vi "WriteData.vi"(8 "error in":errorcluster, 11 "refnum in":refnum<file>) -> (0 "error out":errorcluster, 3 "refnum out":refnum<file>)   [LabVIEW 2017]
doc: "Logs data to csv file on roborio"
uses:
  <vilib>/Rock Robotics/Network Tables/NT Read Number.vi
  <vilib>/Rock Robotics/Network Tables/NT Read Boolean.vi
  <vilib>/Rock Robotics/Network Tables/NT Read String.vi
  Robot Global Data.vi
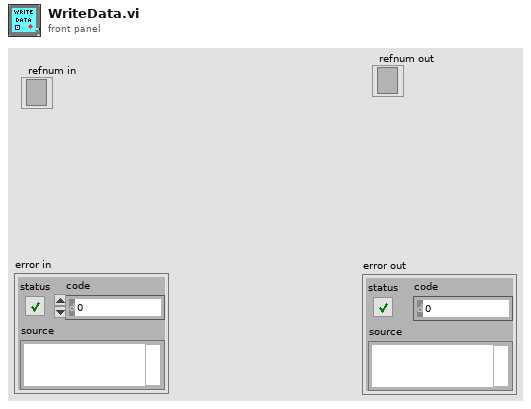
[diagram p1: front panel]
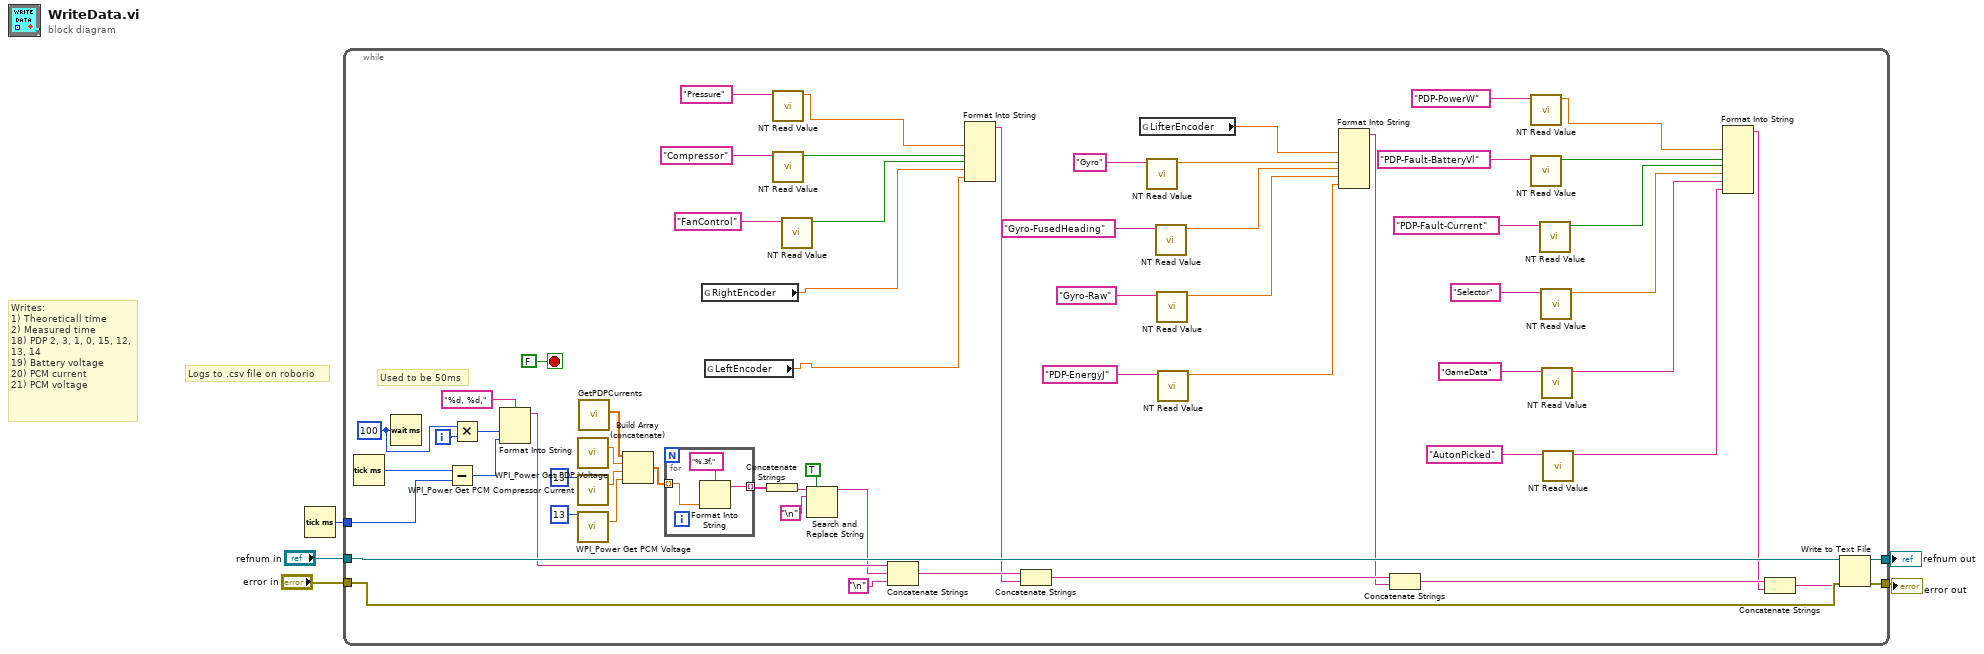
[diagram p0: block diagram]
diagram:
  # "Logs to .csv file on roborio"
  # "Writes:\n1) Theoreticall time\n2) Measured time\n18) PDP 2, 3, 1, 0, 15, 12,\n13, 14\n19) Battery voltage\n20) PCM current\n21) PCM voltage"
  n1 = Tick Count (ms)() -> (millisecond timer value=w1:u32)
  n2 = while {
    tunnel: "error in" -> [w65]
    tunnel: "refnum in" -> [w64]
    tunnel: [w62] -> w3
    tunnel: [w63] -> w2
    tunnel: w1 -> [w61]
    i -> [w66]
    stop <- FALSE stop-if-true
    w60 = u32 100 ("milliseconds to wait")
    # "Used to be 50ms"
    n3 = Tick Count (ms)() -> (millisecond timer value=w48:u32)
    n4 = Wait (ms)(milliseconds to wait=w60) -> ()  [unwired: 1 out]
    n5 = Subtract(x=w48, y=w61) -> (x-y=w47:u32)
    n6 = Multiply(x=w60, y=w66) -> (x*y=w59:u32)
    n7 = Format Into String(format string="%d, %d,", w59, w47) -> (resulting string=w44:string)  [unwired: 2 in, 1 out]
    n8 = call <vilib>:"WPI_Power Get PDP Voltage.vi"() -> ("voltage (V)"=w55:dbl)  [unwired: 14 in, 1 out]
    n9 = call <vilib>:"WPI_Power Get PCM Compressor Current.vi"("Pneumatics Control Module (0)"=u8 13) -> ("current (A)"=w51:dbl)  [unwired: 13 in, 1 out]
    n10 = call <vilib>:"WPI_Power Get PCM Voltage.vi"("Pneumatics Control Module (0)"=u8 13) -> ("Input Voltage"=w50:dbl)  [unwired: 12 in, 2 out]
    n11 = call "GetPDPCurrents.vi"() -> ("PDP Currents"=w49:dbl[])  [unwired: 11 in]
    n12 = Build Array (concatenate)(w49, w55, w51, w50) -> (w54:dbl[])
    n13 = for {
      tunnel: w54 -> [w70] mode=indexing
      tunnel: [w68] -> w53 mode=indexing
      n14 = Format Into String(format string="%.3f,", w70) -> (resulting string=w68:string)  [unwired: 2 in, 1 out]
    }
    n15 = global read "Robot Global Data.vi" "RightEncoder"() -> (w6:dbl)
    n16 = global read "Robot Global Data.vi" "LeftEncoder"() -> (w7:dbl)
    n17 = Concatenate Strings(w53) -> (w52:string)
    n18 = call-poly <vilib>:"NT Read Value.vi"("Name"="Pressure") -> ("Numeric"=w38:dbl)  [unwired: 9 in, 1 out]
    n19 = call-poly <vilib>:"NT Read Value.vi"("Name"="Compressor") -> ("Boolean"=w34:bool)  [unwired: 9 in, 1 out]
    n20 = call-poly <vilib>:"NT Read Value.vi"("Name"="FanControl") -> ("Boolean"=w33:bool)  [unwired: 9 in, 1 out]
    n21 = Search and Replace String(replace all?=TRUE ("replace all? (F)"), input string=w52, search string="\n") -> (result string=w43:string)  [unwired: 5 in, 3 out]
    n22 = Concatenate Strings(w44, w43, "\n") -> (w46:string)
    n23 = Format Into String(w38, w34, w33, w6, w7) -> (resulting string=w39:string)  [unwired: 3 in, 1 out]
    n24 = Concatenate Strings(w46, w39) -> (w40:string)
    n25 = global read "Robot Global Data.vi" "LifterEncoder"() -> (w8:dbl)
    n26 = call-poly <vilib>:"NT Read Value.vi"("Name"="Gyro") -> ("Numeric"=w29:dbl)  [unwired: 9 in, 1 out]
    n27 = call-poly <vilib>:"NT Read Value.vi"("Name"="Gyro-FusedHeading") -> ("Numeric"=w28:dbl)  [unwired: 9 in, 1 out]
    n28 = call-poly <vilib>:"NT Read Value.vi"("Name"="Gyro-Raw") -> ("Numeric"=w27:dbl)  [unwired: 9 in, 1 out]
    n29 = call-poly <vilib>:"NT Read Value.vi"("Name"="PDP-EnergyJ") -> ("Numeric"=w26:dbl)  [unwired: 9 in, 1 out]
    n30 = Format Into String(w8, w29, w28, w27, w26) -> (resulting string=w23:string)  [unwired: 3 in, 1 out]
    n31 = Concatenate Strings(w40, w23) -> (w24:string)
    n32 = call-poly <vilib>:"NT Read Value.vi"("Name"="PDP-PowerW") -> ("Numeric"=w18:dbl)  [unwired: 9 in, 1 out]
    n33 = call-poly <vilib>:"NT Read Value.vi"("Name"="PDP-Fault-BatteryVl") -> ("Boolean"=w19:bool)  [unwired: 9 in, 1 out]
    n34 = call-poly <vilib>:"NT Read Value.vi"("Name"="PDP-Fault-Current") -> ("Boolean"=w20:bool)  [unwired: 9 in, 1 out]
    n35 = call-poly <vilib>:"NT Read Value.vi"("Name"="Selector") -> ("Numeric"=w21:dbl)  [unwired: 9 in, 1 out]
    n36 = call-poly <vilib>:"NT Read Value.vi"("Name"="GameData") -> ("String"=w22:string)  [unwired: 9 in, 1 out]
    n37 = call-poly <vilib>:"NT Read Value.vi"("Name"="AutonPicked") -> ("String"=w9:string)  [unwired: 9 in, 1 out]
    n38 = Format Into String(w18, w19, w20, w21, w22, w9) -> (resulting string=w11:string)  [unwired: 3 in, 1 out]
    n39 = Concatenate Strings(w24, w11) -> (w12:string)
    n40 = Write to Text File(file (use dialog)=w64, text=w12, error in=w65) -> (refnum out=w62:refnum<file>, error out=w63:errorcluster)  [unwired: 1 in, 1 out]
  }
  "refnum out" <- w3
  "error out" <- w2
